vi "Generate Sequence.vi"(8 "error in (no error)":errorcluster, 11 "Maxscend SP4T in":refnum<class "Maxscend SP4T.lvclass">) -> (0 "error out":errorcluster, 3 "Maxscend SP4T out":refnum<class "Maxscend SP4T.lvclass">)   [LabVIEW 2020, in "Maxscend SP4T.lvclass"]
uses:
  Maxscend SP4T.lvclass
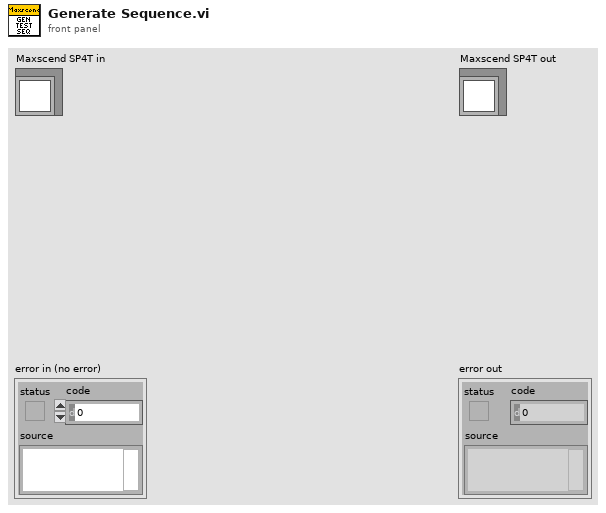
[diagram p1: front panel]
types:
  T1 = cluster{"GPIO Settings":bool[][], "GPIO Values":string[]}
  T2 = enum16{"Vdd", "Control 0", "Control 1", "Control 2", "Control 3"}[]
  T3 = cluster{"Enabled":bool, "State":dbl, "V1 V2 V3":bool[], "RF Path":string}[]
  T4 = typedef "NI DAQmx.lvclass/DAQmx line name.ctl" = cluster{"lines":tag, "Function":string, "Function":enum16{"Vdd", "Control 0", "Control 1", "Control 2", "Control 3"}}
  T5 = enum16{"Vdd", "Control 0", "Control 1", "Control 2", "Control 3"}
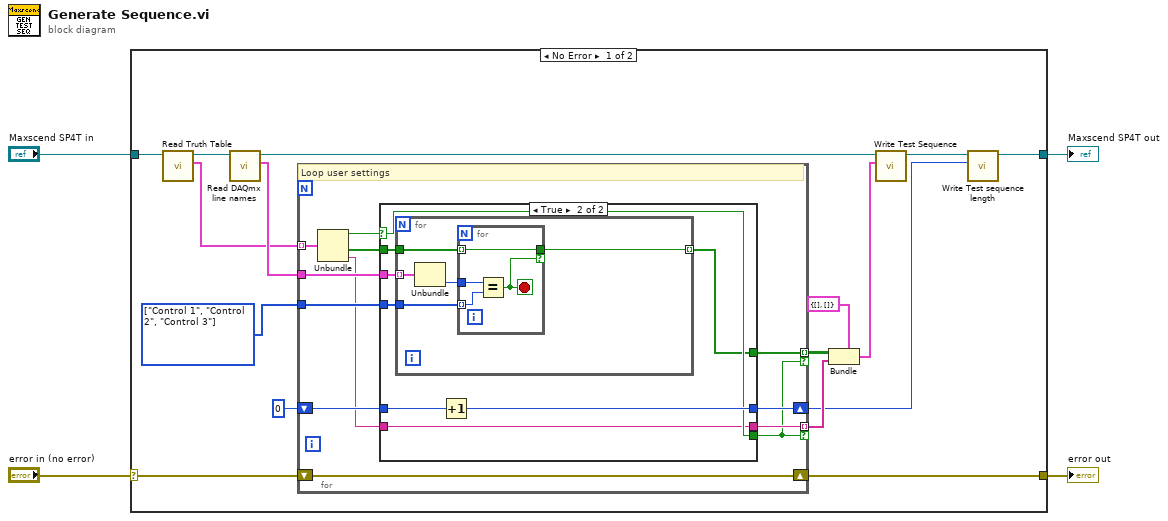
[diagram p0: block diagram]
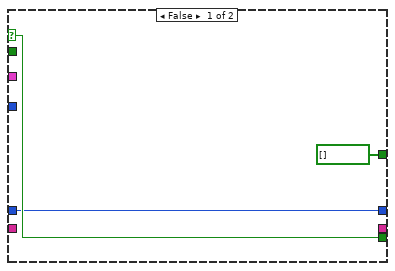
[diagram p2: hidden frame]
diagram:
  n1 = case shown="No Error" "error in (no error)" {
    selector: "error in (no error)" -> [w20 w54]
    tunnel: [w19 w54] -> w3
    tunnel: [w7 w53] -> w1
    tunnel: "Maxscend SP4T in" -> [w16 w53]
    frame No Error {
      w13 = T2 [enum."Control 1", enum."Control 2", enum."Control 3"] items=["Vdd", "Control 0", "Control 1", "Control 2", "Control 3"]
      n2 = call-dynamic "Read Truth Table.vi"("Maxscend SP4T in"=w16) -> ("Truth Table"=w14:T3, "Maxscend SP4T out"=w15:refnum<class "Maxscend SP4T.lvclass">)  [unwired: 9 in]
      n3 = call-dynamic "Read DAQmx line names.vi"("NI DAQmx in"=w15) -> ("DAQmx line names"=w18:T4[], "NI DAQmx out"=w17:refnum<class "Maxscend SP4T.lvclass">)  [unwired: 8 in, 1 out]
      n4 = for {
        tunnel: w14 -> [w26] mode=indexing
        tunnel: w18 -> [w32]
        tunnel: w13 -> [w31]
        shift-right: [w29] -> w5
        shift-left: 0 ("Test sequence length") -> [w30]
        tunnel: [w28] -> w10 mode=indexing if=w21
        tunnel: [w27] -> w9 mode=indexing if=w21
        shift-right: [w23] -> w19
        shift-left: w20 -> [w23]
        # "Loop user settings"
        n5 = Unbundle(w26) -> ("Enabled"=w25:bool, "V1 V2 V3"=w24:bool[], "RF Path"=w22:string)  [unwired: 1 out]
        n6 = case shown="True" w25 {
          selector: w25 -> [w35 w38]
          tunnel: w32 -> [_ w43]
          tunnel: w31 -> [_ w42]
          tunnel: w24 -> [_ w41]
          tunnel: w30 -> [w34 w40]
          tunnel: [w34 w39] -> w29
          tunnel: [_ w36] -> w28
          tunnel: [w35 w38] -> w21
          tunnel: [bool[] [] w37] -> w27
          tunnel: w22 -> [_ w36]
          frame False {
          }
          frame True {
            n7 = for {
              tunnel: w43 -> [w48] mode=indexing
              tunnel: w42 -> [w47]
              tunnel: w41 -> [w45]
              tunnel: [w44] -> w37 mode=indexing
              n8 = Unbundle(w48) -> ("Function"=w46:T5)  [unwired: 2 out]
              n9 = for {
                tunnel: w47 -> [w51] mode=indexing
                tunnel: w46 -> [w52]
                tunnel: w45 -> [w50] mode=indexing
                tunnel: [w50] -> w44 if=w49
                stop <- w49 stop-if-true
                n10 = Equal?(x=w52, y=w51) -> (x = y?=w49:bool)
              }
            }
            n11 = Increment(x=w40) -> (x+1=w39:i32)
          }
        }
      }
      n12 = Bundle(cluster=T1 {"GPIO Settings"=[], "GPIO Values"=[]} ("Test Sequence"), "GPIO Settings"=w9, "GPIO Values"=w10) -> (w11:T1)
      n13 = call-dynamic "Write Test Sequence.vi"("Test Sequence"=w11, "NI DAQmx in"=w17) -> ("NI DAQmx out"=w8:refnum<class "Maxscend SP4T.lvclass">)  [unwired: 8 in, 1 out]
      n14 = call-dynamic "Write Test sequence length.vi"("Test sequence length"=w5, "Device in"=w8) -> ("Device out"=w7:refnum<class "Maxscend SP4T.lvclass">)  [unwired: 8 in, 1 out]
    }
    frame Error {
    }
  }
  "error out" <- w3
  "Maxscend SP4T out" <- w1
